vi "test Connect.vi"(8 "error in (no error)":errorcluster, 11 "TestCase in":refnum<class "Test Network Stream Listener Connect.lvclass">) -> (0 "error out":errorcluster, 3 "TestCase out":refnum<class "Test Network Stream Listener Connect.lvclass">)   [LabVIEW 2020, in "Test Network Stream Listener Connect.lvclass"]
uses:
  Test Network Stream Listener Connect.lvclass
  <vilib>/addons/_JKI Toolkits/VI Tester/TestCase.llb/TestCase.lvclass
  Source/Protocols/Network Stream Strategy/Netowrk Stream Listener/Network Stream Listener.lvclass
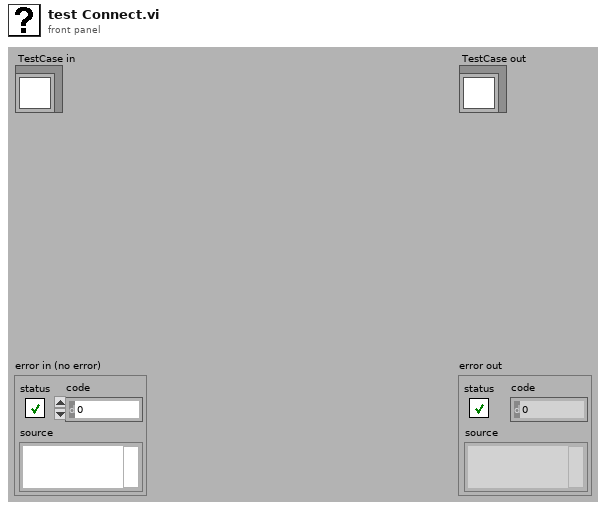
[diagram p1: front panel]
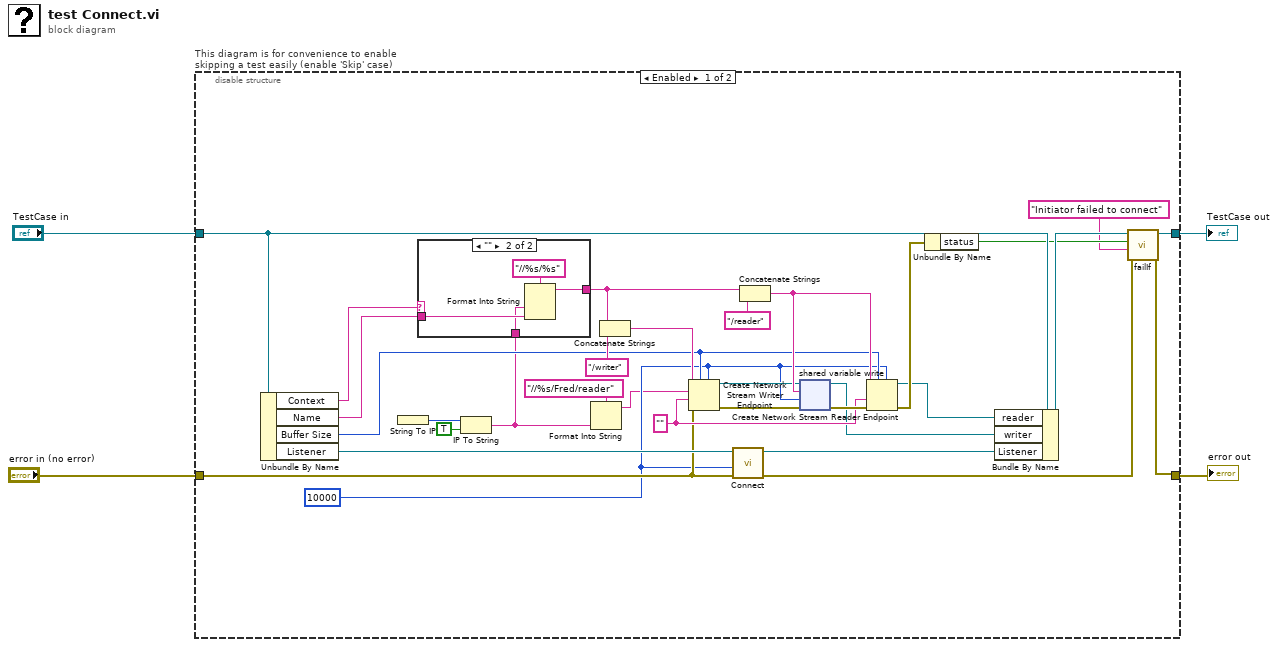
[diagram p0: block diagram]
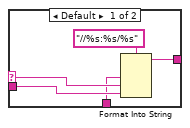
[diagram p2: hidden frame]
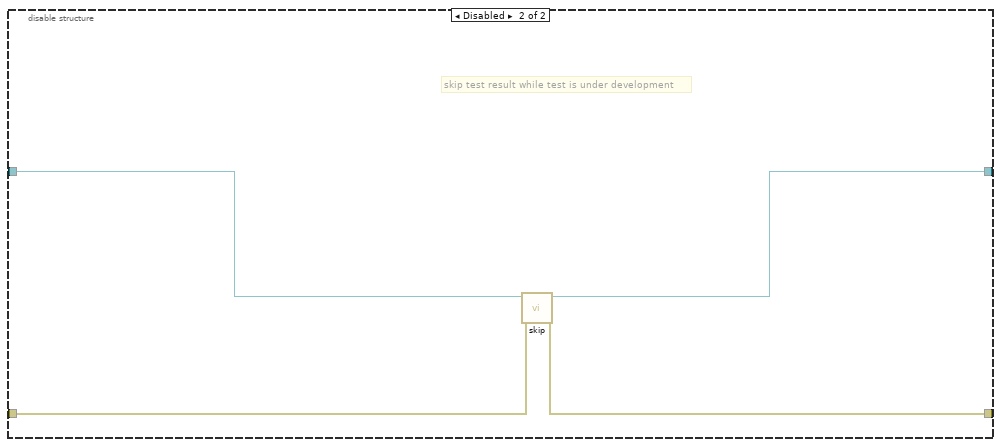
[diagram p3: hidden frame]
diagram:
  n1 = disable-structure "This diagram is for convenience to enable skipping a test easily (enable 'Skip' case)" shown="Enabled" {
    disable-tunnel: "TestCase in" -> [w31 w48]
    disable-tunnel: [w35 w46] -> w1
    disable-tunnel: [w34 w47] -> w3
    disable-tunnel: "error in (no error)" -> [w17 w45]
    frame Enabled {
      w18 = ""
      w11 = 10000 ("timeout")
      n2 = Unbundle By Name(w31) -> ("Context"=w14:string, "Name"=w13:string, "Buffer Size"=w12:i32, "Listener"=w32:refnum<class "Network Stream Listener.lvclass">)
      n3 = String To IP() -> (0:w16:u32)  [unwired: 1 in]
      n4 = IP To String(1:TRUE ("dot notation? (F)"), 2:w16) -> (0:w7:string)
      n5 = case shown="\"\"" w14 {
        selector: w14 -> [w37 _]
        tunnel: [w39 w44] -> w22
        tunnel: w13 -> [w38 w42]
        tunnel: w7 -> [w36 w41]
        frame Default {
          n6 = Format Into String(format string="//%s:%s/%s", w36, w37, w38) -> (resulting string=w39:string)  [unwired: 2 in, 1 out]
        }
        frame "" {
          n7 = Format Into String(format string="//%s/%s", w41, w42) -> (resulting string=w44:string)  [unwired: 2 in, 1 out]
        }
      }
      n8 = Format Into String(format string="//%s/Fred/reader", w7) -> (resulting string=w5:string)  [unwired: 2 in, 1 out]
      n9 = Concatenate Strings(w22, "/writer" ("format string")) -> (w20:string)
      n10 = Create Network Stream Writer Endpoint(5:w11, 7:w12, 8:w17, 9:w18, 10:w5, 11:w20) -> (0:w23:errorcluster, 3:w25:refnum<k21>)  [unwired: 1 in]
      n11 = call-dynamic "Connect.vi"("error in (no error)"=w17, "timeout"=w11, "Network Stream in"=w32) -> ("error out"=w33:errorcluster, "Network Stream out"=w29:refnum<class "Network Stream Listener.lvclass">)  [unwired: 7 in]
      n12 = Concatenate Strings(w22, "/reader" ("format string")) -> (w26:string)
      n13 = shared-variable-write(w25, w23, w26, w11) -> (w8:refnum<k21>, w24:errorcluster)  [unwired: 1 out]
      n14 = Create Network Stream Reader Endpoint(5:w11, 7:w12, 8:w24, 9:w18, 11:w26) -> (0:w10:errorcluster, 3:w9:refnum<k21>)  [unwired: 2 in]
      n15 = Unbundle By Name(w10) -> ("status"=w28:bool)
      n16 = Bundle By Name(cluster=w31, "reader"=w9, "writer"=w8, "Listener"=w29) -> (w30:refnum<class "Test Network Stream Listener Connect.lvclass">)
      n17 = call-dynamic "failIf.vi"("error in (no error)"=w33, "message (\"\")"="Initiator failed to connect" ("message (\"\")"), "fail"=w28, "TestCase in"=w30) -> ("error out"=w34:errorcluster, "TestCase out"=w35:refnum<class "Test Network Stream Listener Connect.lvclass">)  [unwired: 6 in]
    }
    frame Disabled {
      # "skip test result while test is under development"
      n18 = call <vilib>:"skip.vi"("error in (no error)"=w45, "TestCase in"=w48) -> ("error out"=w47:errorcluster, "TestCase out"=w46:refnum<class "Test Network Stream Listener Connect.lvclass">)  [unwired: 8 in]
    }
  }
  "error out" <- w3
  "TestCase out" <- w1
